vi "Right To Near Rocket From Feeder Station.vi"   [LabVIEW 2018]
uses:
  Framework/Robot Global Data.vi
  Support Code/Path Data.ctl
types:
  T1 = typedef "Command Status Info.ctl" = cluster{"Name":string, "Status":T2, "notifier out":T3}
  T2 = typedef "Completion Status.ctl" = enum16{"Successful", "Aborted", "Incomplete"}
  T3 = typedef "Completion Notifier.ctl" = refnum<notifier>
  T4 = typedef "Path Data.ctl" = cluster{"Maneuver":enum16{"MAX 90", "MAX 180", "Turn to Home", "Turn to Rocket", "Auto-Align", "Turn to ..."}, "Rotation Direction":enum16{"N/A", "Right", "Left"}}[]
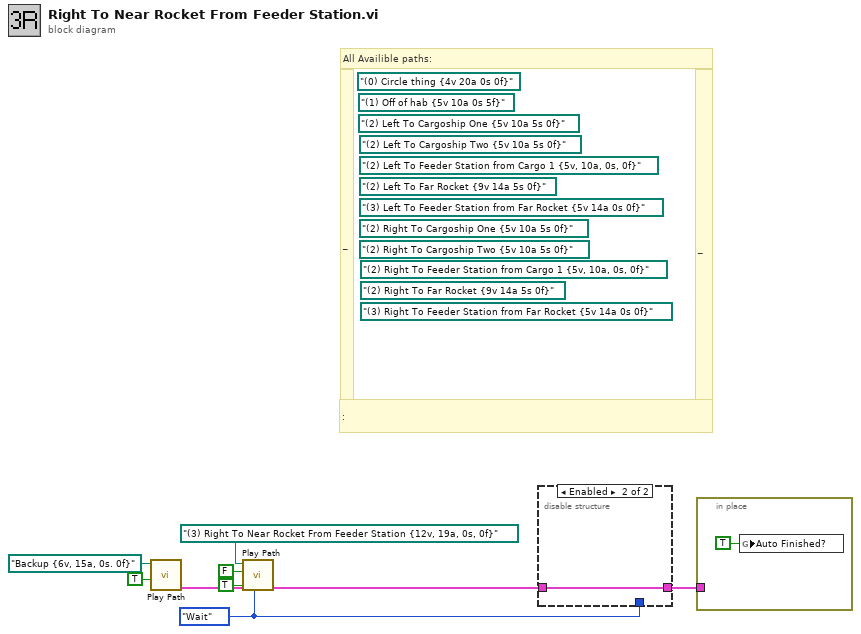
[diagram p0: block diagram]
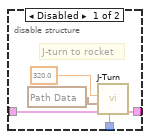
[diagram p2: hidden frame]
diagram:
  (unwired) path "(3) Right To Feeder Station from Far Rocket {5v 14a 0s 0f}"
  (unwired) path "(2) Right To Far Rocket {9v 14a 5s 0f}"
  (unwired) path "(2) Right To Feeder Station from Cargo 1 {5v, 10a, 0s, 0f}"
  (unwired) path "(2) Right To Cargoship Two {5v 10a 5s 0f}"
  (unwired) path "(2) Right To Cargoship One {5v 10a 5s 0f}"
  (unwired) path "(3) Left To Feeder Station from Far Rocket {5v 14a 0s 0f}"
  (unwired) path "(2) Left To Far Rocket {9v 14a 5s 0f}"
  (unwired) path "(2) Left To Feeder Station from Cargo 1 {5v, 10a, 0s, 0f}"
  (unwired) path "(2) Left To Cargoship Two {5v 10a 5s 0f}"
  (unwired) path "(2) Left To Cargoship One {5v 10a 5s 0f}"
  (unwired) path "(1) Off of hab {5v 10a 0s 5f}"
  w5 = enum16{"Start", "Wait"}."Wait" ("Synchronication")
  (unwired) path "(0) Circle thing {4v 20a 0s 0f}"
  # ":"
  # "_"
  # "_"
  # "All Availible paths:"
  n1 = call "Play Path.vi"("Reverse (T) / Normal (F)"=TRUE, "Path"=path "Backup {6v, 15a, 0s. 0f}") -> ("Command Info Out"=w3:T1)  [unwired: 9 in]
  n2 = call "Play Path.vi"("Synchronication"=w5, "Command Info In"=w3, "Reverse (T) / Normal (F)"=TRUE, "Path Reversed"=FALSE, "Path"=path "(3) Right To Near Rocket From Feeder Station {12v, 19a, 0s, 0f}") -> ("Command Info Out"=w4:T1)  [unwired: 6 in]
  n3 = disable-structure shown="Enabled" {
    disable-tunnel: [w13 w15] -> w8
    disable-tunnel: w5 -> [w11 _]
    disable-tunnel: w4 -> [w10 w15]
    frame Disabled {
      # "J-turn to rocket"
      n4 = call "J-Turn.vi"("Synchronication"=w11, "Command Info In"=w10, "Path Data"=T4 [{"Maneuver"=enum."Turn to ...", "Rotation Direction"=enum."N/A"}, {"Maneuver"=enum."MAX 90", "Rotation Direction"=enum."N/A"}, {"Maneuver"=enum."MAX 90", "Rotation Direction"=enum."N/A"}], "Angle boi"=320.0) -> ("Command Info Out"=w13:T1)  [unwired: 7 in]
    }
    frame Enabled {
    }
  }
  n5 = in-place {
    in-place-border: w8 -> [_]
    n6 = global write "Robot Global Data.vi" "Auto Finished?"(TRUE ("Auto Finished?")) -> ()
  }
